vi "sv_Get Chirp Waveform Attribute.vi"(8 "error in (no error)":errorcluster, 10 "chirp attributes":T1(ring), 11 "chirp signal":waveform(dbl)={"t0"=timestamp(0 s since 1904-01-01), "dt"=0.0, "Y"=[]}) -> (0 "error out":errorcluster, 2 "attribute value":variant, 3 "chirp signal out":waveform(dbl))   [LabVIEW 2017, in "SoundVib_Generation.lvlib"]
uses:
  <vilib>/addons/_NISVFA/_Generation/SoundVib_Generation.lvlib
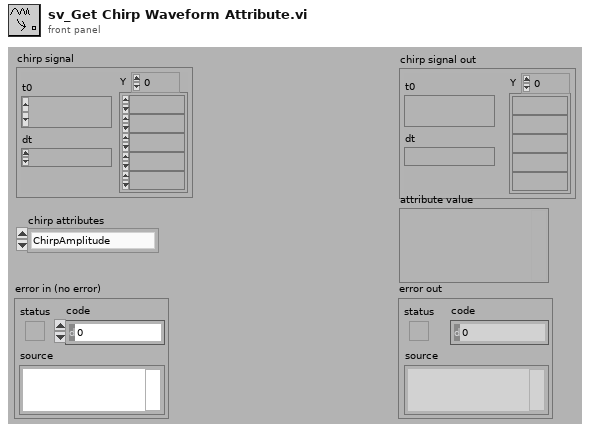
[diagram p1: front panel]
types:
  T1 = enum16{"ChirpAmplitude", "ChirpStartFrequency", "ChirpStopFrequency", "ChirpFrequencySpacing", "ChirpSamplingRate", "ChirpDuration", "ChirpCurrentFrequency", "ChirpCurrentPhase", "ChirpCurrentTime", "ChirpSlope", "ChirpMaxHarmonic", "ChirpPrefixInteger", "ChirpPrefixFractional"}
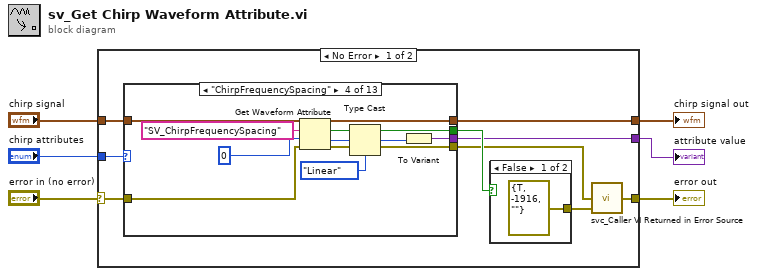
[diagram p0: block diagram]
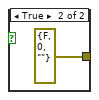
[diagram p2: hidden frame]
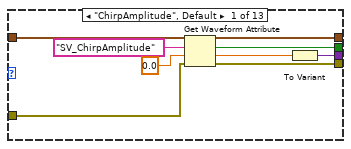
[diagram p3: hidden frame]
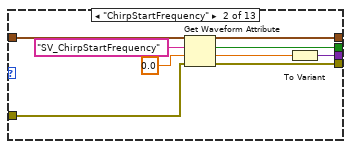
[diagram p4: hidden frame]
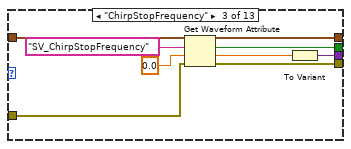
[diagram p5: hidden frame]
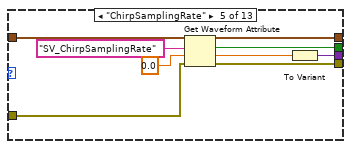
[diagram p6: hidden frame]
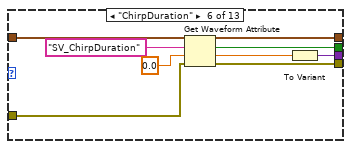
[diagram p7: hidden frame]
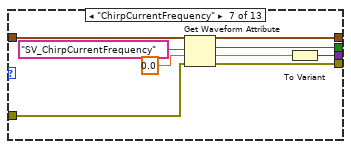
[diagram p8: hidden frame]
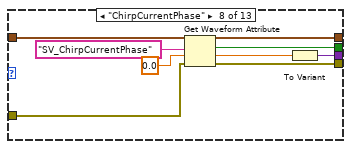
[diagram p9: hidden frame]
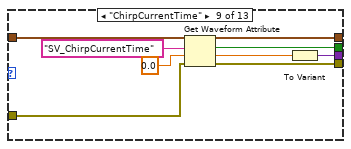
[diagram p10: hidden frame]
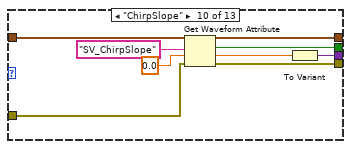
[diagram p11: hidden frame]
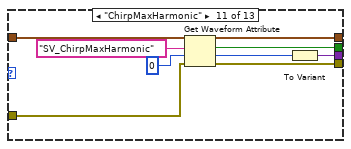
[diagram p12: hidden frame]
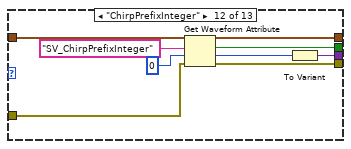
[diagram p13: hidden frame]
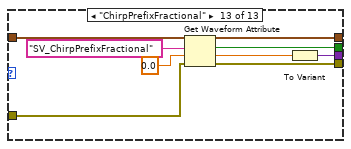
[diagram p14: hidden frame]
diagram:
  n1 = case shown="No Error" "error in (no error)" {
    selector: "error in (no error)" -> [w13 w138]
    tunnel: "chirp signal" -> [w15 w137]
    tunnel: [w7 w138] -> w4
    tunnel: [w9 w137] -> w3
    tunnel: "chirp attributes" -> [w14 _]
    tunnel: [w8 _] -> w1
    frame No Error {
      n2 = case shown="\"ChirpFrequencySpacing\"" w14 {
        tunnel: w15 -> [w26 w35 w44 w55 w64 w73 w82 w91 w100 w109 w118 w127 w136]
        tunnel: [w22 w32 w41 w54 w61 w70 w79 w88 w97 w106 w115 w124 w133] -> w8
        tunnel: w13 -> [w19 w29 w38 w51 w58 w67 w76 w85 w94 w103 w112 w121 w130]
        tunnel: [w21 w31 w40 w53 w60 w69 w78 w87 w96 w105 w114 w123 w132] -> w12
        tunnel: [w20 w30 w39 w52 w59 w68 w77 w86 w95 w104 w113 w122 w131] -> w9
        tunnel: [w18 w27 w36 w49 w56 w65 w74 w83 w92 w101 w110 w119 w128] -> w10
        frame "ChirpAmplitude", Default {
          n3 = Get Waveform Attribute(4:w19, 5:0.0, 6:"SV_ChirpAmplitude" ("name"), 7:w26) -> (0:w18:errorcluster, 1:w23:dbl, 2:w21:bool, 3:w20:waveform(dbl))
          n4 = To Variant(anything=w23) -> (Variant=w22:variant)
        }
        frame "ChirpStartFrequency" {
          n5 = Get Waveform Attribute(4:w29, 5:0.0, 6:"SV_ChirpStartFrequency" ("name"), 7:w35) -> (0:w27:errorcluster, 1:w33:dbl, 2:w31:bool, 3:w30:waveform(dbl))
          n6 = To Variant(anything=w33) -> (Variant=w32:variant)
        }
        frame "ChirpStopFrequency" {
          n7 = Get Waveform Attribute(4:w38, 5:0.0, 6:"SV_ChirpStopFrequency" ("name"), 7:w44) -> (0:w36:errorcluster, 1:w42:dbl, 2:w40:bool, 3:w39:waveform(dbl))
          n8 = To Variant(anything=w42) -> (Variant=w41:variant)
        }
        frame "ChirpFrequencySpacing" {
          n9 = Get Waveform Attribute(4:w51, 5:u16 0, 6:"SV_ChirpFrequencySpacing" ("name"), 7:w55) -> (0:w49:errorcluster, 1:w47:u16, 2:w53:bool, 3:w52:waveform(dbl))
          n10 = Type Cast(type=enum16{"Linear", "Logarithmic"}."Linear" ("frequency range.frequency spacing"), x=w47) -> (*(type *) &x=w46:enum16{"Linear", "Logarithmic"})
          n11 = To Variant(anything=w46) -> (Variant=w54:variant)
        }
        frame "ChirpSamplingRate" {
          n12 = Get Waveform Attribute(4:w58, 5:0.0, 6:"SV_ChirpSamplingRate" ("name"), 7:w64) -> (0:w56:errorcluster, 1:w62:dbl, 2:w60:bool, 3:w59:waveform(dbl))
          n13 = To Variant(anything=w62) -> (Variant=w61:variant)
        }
        frame "ChirpDuration" {
          n14 = Get Waveform Attribute(4:w67, 5:0.0, 6:"SV_ChirpDuration" ("name"), 7:w73) -> (0:w65:errorcluster, 1:w71:dbl, 2:w69:bool, 3:w68:waveform(dbl))
          n15 = To Variant(anything=w71) -> (Variant=w70:variant)
        }
        frame "ChirpCurrentFrequency" {
          n16 = Get Waveform Attribute(4:w76, 5:0.0, 6:"SV_ChirpCurrentFrequency" ("name"), 7:w82) -> (0:w74:errorcluster, 1:w80:dbl, 2:w78:bool, 3:w77:waveform(dbl))
          n17 = To Variant(anything=w80) -> (Variant=w79:variant)
        }
        frame "ChirpCurrentPhase" {
          n18 = Get Waveform Attribute(4:w85, 5:0.0, 6:"SV_ChirpCurrentPhase" ("name"), 7:w91) -> (0:w83:errorcluster, 1:w89:dbl, 2:w87:bool, 3:w86:waveform(dbl))
          n19 = To Variant(anything=w89) -> (Variant=w88:variant)
        }
        frame "ChirpCurrentTime" {
          n20 = Get Waveform Attribute(4:w94, 5:0.0, 6:"SV_ChirpCurrentTime" ("name"), 7:w100) -> (0:w92:errorcluster, 1:w98:dbl, 2:w96:bool, 3:w95:waveform(dbl))
          n21 = To Variant(anything=w98) -> (Variant=w97:variant)
        }
        frame "ChirpSlope" {
          n22 = Get Waveform Attribute(4:w103, 5:0.0, 6:"SV_ChirpSlope" ("name"), 7:w109) -> (0:w101:errorcluster, 1:w107:dbl, 2:w105:bool, 3:w104:waveform(dbl))
          n23 = To Variant(anything=w107) -> (Variant=w106:variant)
        }
        frame "ChirpMaxHarmonic" {
          n24 = Get Waveform Attribute(4:w112, 5:0, 6:"SV_ChirpMaxHarmonic" ("name"), 7:w118) -> (0:w110:errorcluster, 1:w116:i32, 2:w114:bool, 3:w113:waveform(dbl))
          n25 = To Variant(anything=w116) -> (Variant=w115:variant)
        }
        frame "ChirpPrefixInteger" {
          n26 = Get Waveform Attribute(4:w121, 5:u32 0, 6:"SV_ChirpPrefixInteger" ("name"), 7:w127) -> (0:w119:errorcluster, 1:w125:u32, 2:w123:bool, 3:w122:waveform(dbl))
          n27 = To Variant(anything=w125) -> (Variant=w124:variant)
        }
        frame "ChirpPrefixFractional" {
          n28 = Get Waveform Attribute(4:w130, 5:0.0, 6:"SV_ChirpPrefixFractional" ("name"), 7:w136) -> (0:w128:errorcluster, 1:w134:dbl, 2:w132:bool, 3:w131:waveform(dbl))
          n29 = To Variant(anything=w134) -> (Variant=w133:variant)
        }
      }
      n30 = case shown="False" w12 {
        tunnel: [errorcluster {"status"=TRUE, "code"=-1916, "source"=""} ("error in (no error)") errorcluster {"status"=FALSE, "code"=0, "source"=""} ("error in (no error)")] -> w11
        frame False {
        }
        frame True {
        }
      }
      n31 = call <vilib>:"svc_Caller VI Returned in Error Source.vi"("warning input to caller"=w11, "error in (no error)"=w10) -> ("error out"=w7:errorcluster)  [unwired: 3 in]
    }
    frame Error {
    }
  }
  "error out" <- w4
  "chirp signal out" <- w3
  "attribute value" <- w1
